vi "Lakeshore_372_write.vi"(5 "File reference":refnum<file>) -> ()   [LabVIEW 2019]
uses:
  Instrument_Setup.vi
  Global/Global Variables/Data_Display_global.vi
  Global/Global Variables/global.vi
panel:
  # "OFF"
  # "ON"
  # "OFF"
  # "ON"
  # "OFF"
  # "ON"
  # "OFF"
  # "ON"
  # "ON"
  # "OFF"
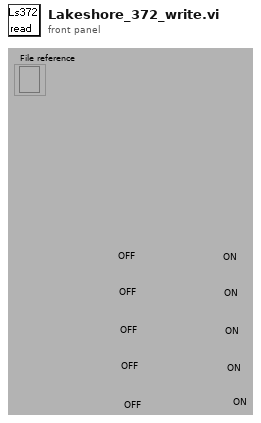
[diagram p1: front panel]
types:
  T1 = typedef "LS372-Cluster.ctl" = cluster{"Activate Tsweep":bool, "Setpoint - Manual":dbl, "Rate (K/min)":dbl, "Update Lakeshores":bool, "Still Heater":bool, "Still Power (mW)":dbl, "Manual Heater":bool, "Manual Heater  (mW) ":dbl, "Heater Range":dbl, "P (Gain)":dbl, "I (Reset)":dbl, "D (Rate)":dbl, "Heater Power (mW)":dbl, "MC Thermometer":u16, "MC Temperature":dbl, "LS372-T1":dbl, "LS372 -T2":dbl, "LS372-R1 ":dbl, "LS372-R2":dbl, "LS372-T3":dbl, "LS372-T4":dbl, "LS372-R3 ":dbl, "LS372-R4 \n\n\n\n":dbl, "LS372-T5":dbl, "LS372-T6":dbl, "LS372-R5":dbl, "LS372-R6 ":dbl, "Still Power ist":dbl, "Set Temperatur Sweep main":bool, "Setpoint ist":dbl, "Disable Heater":bool}
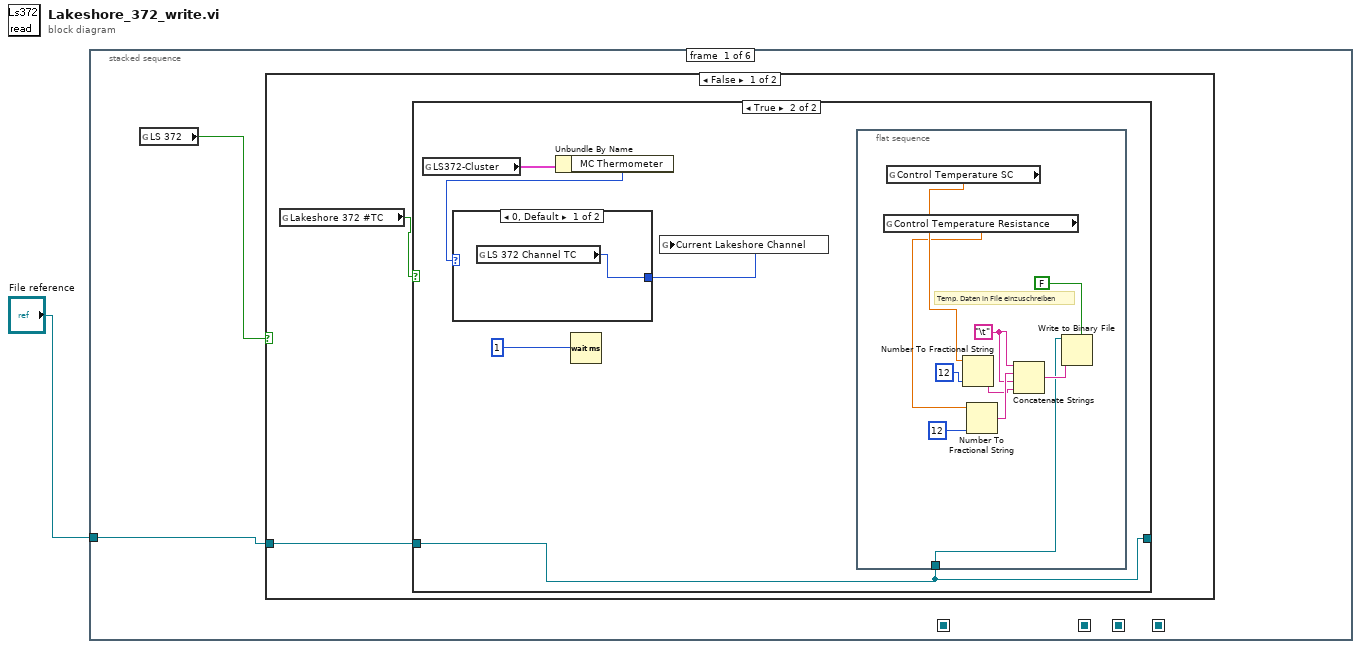
[diagram p0: block diagram]
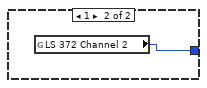
[diagram p3: hidden frame]
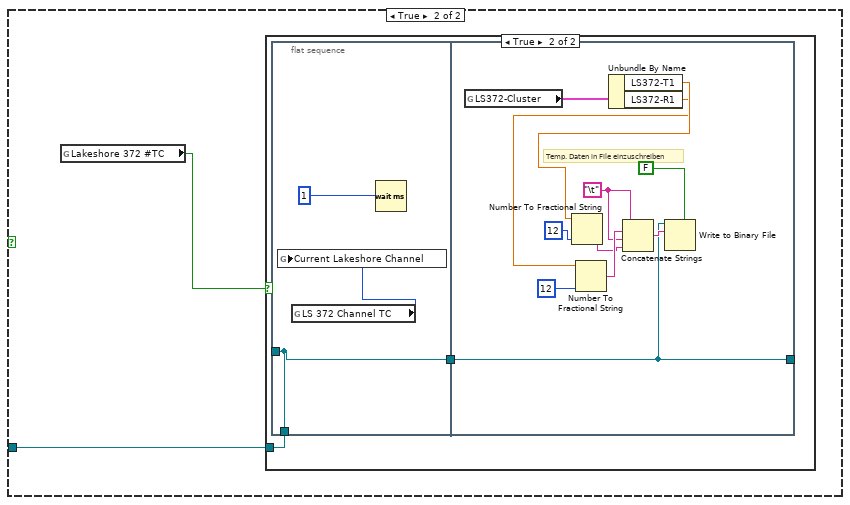
[diagram p4: hidden frame]
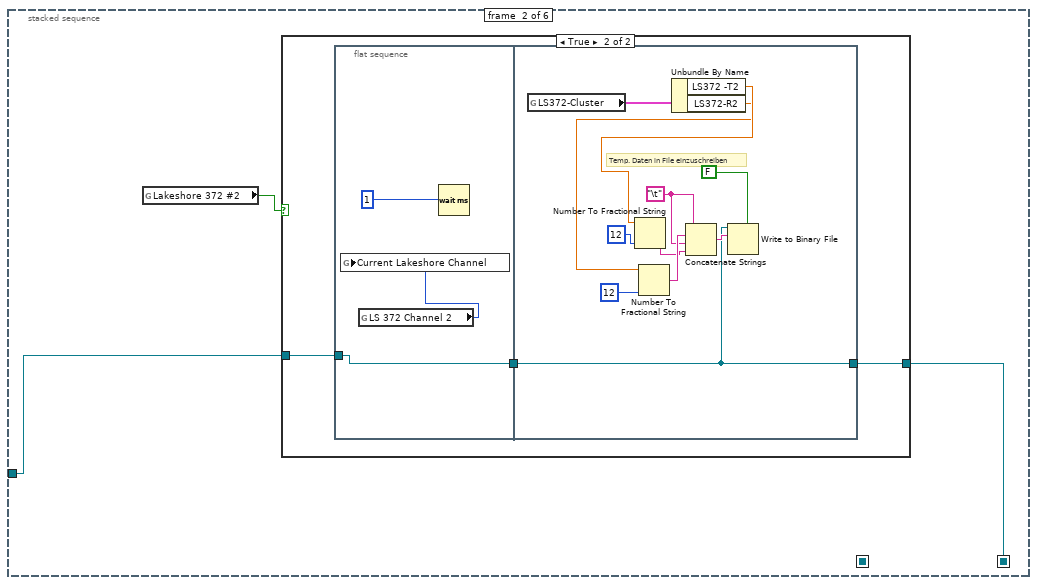
[diagram p6: hidden frame]
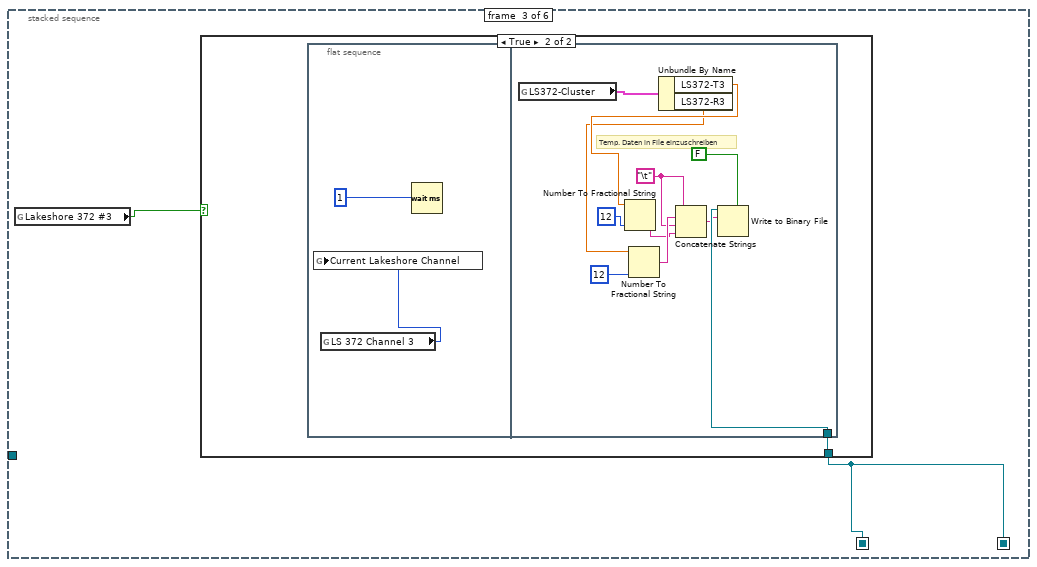
[diagram p8: hidden frame]
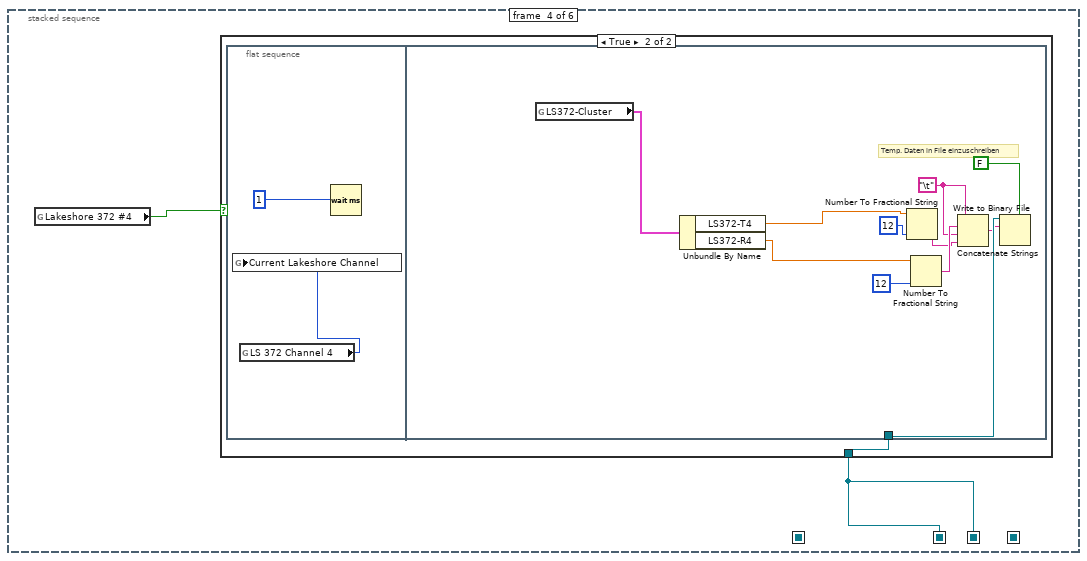
[diagram p10: hidden frame]
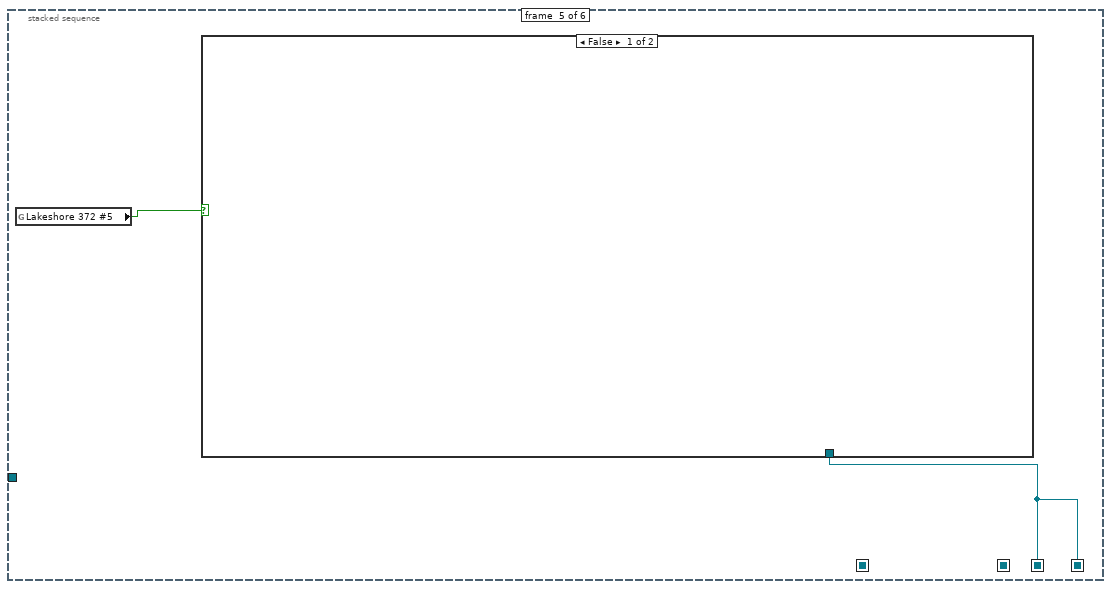
[diagram p12: hidden frame]
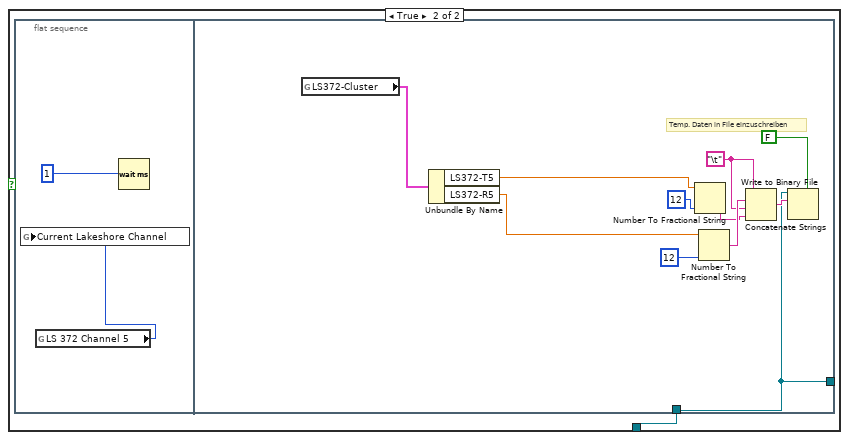
[diagram p13: hidden frame]
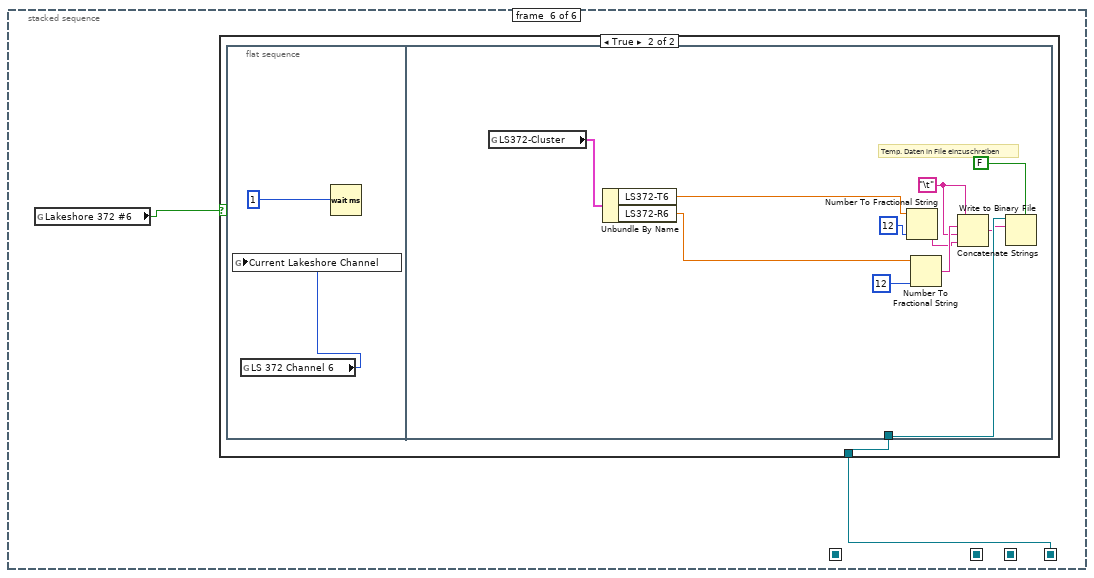
[diagram p14: hidden frame]
diagram:
  n1 = stacked-sequence {
    seq-local: [_ w42 _ _ _ _] -> [_ _ w63 w79 _ _]
    seq-local: [_ _ w63 _ _ _] -> [_ _ _ _ _ _]
    seq-local: [_ _ _ w79 _ _] -> [_ _ _ _ w95 _]
    seq-local: [_ _ _ _ w95 _] -> [_ _ _ _ _ w111]
    tunnel: "File reference" -> [w3 w43 _ _ _ _]
    frame #0 {
      n2 = global read "Instrument_Setup.vi" "LS 372"() -> (w2:bool)
      n3 = case shown="False" w2 {
        tunnel: w3 -> [w4 w24]
        frame False {
          n4 = global read "Instrument_Setup.vi" "Lakeshore 372 #TC"() -> (w5:bool)
          n5 = case shown="True" w5 {
            tunnel: w4 -> [w6 w7]
            tunnel: [w6 w7] -> _
            frame False {
            }
            frame True {
              n6 = global read "Data_Display_global.vi" "LS372-Cluster"() -> (w10:T1)
              n7 = Unbundle By Name(w10) -> ("MC Thermometer"=w9:u16)
              n8 = case shown="0, Default" w9 {
                tunnel: [w12 w13] -> w8
                frame 0, Default {
                  n9 = global read "Instrument_Setup.vi" "LS 372 Channel TC"() -> (w12:u16)
                }
                frame 1 {
                  n10 = global read "Instrument_Setup.vi" "LS 372 Channel 2"() -> (w13:u16)
                }
              }
              n11 = Wait (ms)(milliseconds to wait=1) -> ()  [unwired: 1 out]
              n12 = global write "global.vi" "Current Lakeshore Channel"(w8) -> ()
              n13 = flat-sequence {
                tunnel: w7 -> [w19]
                frame #0 {
                  w17 = "\t"
                  # "Temp. Daten in File einzuschreiben"
                  n14 = global read "Data_Display_global.vi" "Control Temperature Resistance"() -> (w14:dbl)
                  n15 = global read "Data_Display_global.vi" "Control Temperature SC"() -> (w15:dbl)
                  n16 = Number To Fractional String(number=w15, precision (6)=i16 12) -> (F-format string=w16:string)  [unwired: 2 in]
                  n17 = Number To Fractional String(number=w14, precision (6)=i16 12) -> (F-format string=w22:string)  [unwired: 2 in]
                  n18 = Concatenate Strings(w17, w22, w17, w16) -> (w23:string)
                  n19 = Write to Binary File ("Write File")(file (use dialog)=w19, data=w23, 5:FALSE ("prepend array or string size? (T)")) -> ()  [unwired: 3 in, 3 out]
                }
              }
            }
          }
        }
        frame True {
          n20 = global read "Instrument_Setup.vi" "Lakeshore 372 #TC"() -> (w25:bool)
          n21 = case shown="True" w25 {
            tunnel: w24 -> [_ w26]
            frame False {
            }
            frame True {
              n22 = flat-sequence {
                tunnel: [w28] -> _
                tunnel: [w28] -> w27
                tunnel: w26 -> [w28]
                tunnel: w27 -> [w34]
                tunnel: [w34] -> _
                frame #0 {
                  n23 = global read "Instrument_Setup.vi" "LS 372 Channel TC"() -> (w29:u16)
                  n24 = global write "global.vi" "Current Lakeshore Channel"(w29) -> ()
                  n25 = Wait (ms)(milliseconds to wait=1) -> ()  [unwired: 1 out]
                }
                frame #1 {
                  w37 = "\t"
                  # "Temp. Daten in File einzuschreiben"
                  n26 = global read "Data_Display_global.vi" "LS372-Cluster"() -> (w33:T1)
                  n27 = Unbundle By Name(w33) -> ("LS372-T1"=w32:dbl, "LS372-R1"=w31:dbl)
                  n28 = Number To Fractional String(number=w32, precision (6)=i16 12) -> (F-format string=w36:string)  [unwired: 2 in]
                  n29 = Number To Fractional String(number=w31, precision (6)=i16 12) -> (F-format string=w40:string)  [unwired: 2 in]
                  n30 = Concatenate Strings(w37, w40, w37, w36) -> (w35:string)
                  n31 = Write to Binary File ("Write File")(file (use dialog)=w34, data=w35, 5:FALSE ("prepend array or string size? (T)")) -> ()  [unwired: 3 in, 3 out]
                }
              }
            }
          }
        }
      }
    }
    frame #1 {
      n32 = global read "Instrument_Setup.vi" "Lakeshore 372 #2"() -> (w44:bool)
      n33 = case shown="True" w44 {
        tunnel: w43 -> [w45 w48]
        tunnel: [w45 w46] -> w42
        frame False {
        }
        frame True {
          n34 = flat-sequence {
            tunnel: w48 -> [w49]
            tunnel: [w49] -> w47
            tunnel: w47 -> [w55]
            tunnel: [w55] -> w46
            frame #0 {
              n35 = global read "Instrument_Setup.vi" "LS 372 Channel 2"() -> (w50:u16)
              n36 = global write "global.vi" "Current Lakeshore Channel"(w50) -> ()
              n37 = Wait (ms)(milliseconds to wait=1) -> ()  [unwired: 1 out]
            }
            frame #1 {
              w58 = "\t"
              # "Temp. Daten in File einzuschreiben"
              n38 = global read "Data_Display_global.vi" "LS372-Cluster"() -> (w54:T1)
              n39 = Unbundle By Name(w54) -> ("LS372 -T2"=w53:dbl, "LS372-R2"=w52:dbl)
              n40 = Number To Fractional String(number=w53, precision (6)=i16 12) -> (F-format string=w57:string)  [unwired: 2 in]
              n41 = Number To Fractional String(number=w52, precision (6)=i16 12) -> (F-format string=w61:string)  [unwired: 2 in]
              n42 = Concatenate Strings(w58, w61, w58, w57) -> (w56:string)
              n43 = Write to Binary File ("Write File")(file (use dialog)=w55, data=w56, 5:FALSE ("prepend array or string size? (T)")) -> ()  [unwired: 3 in, 3 out]
            }
          }
        }
      }
    }
    frame #2 {
      n44 = global read "Instrument_Setup.vi" "Lakeshore 372 #3"() -> (w64:bool)
      n45 = case shown="True" w64 {
        tunnel: w63 -> [_ w65]
        frame False {
        }
        frame True {
          n46 = flat-sequence {
            tunnel: w65 -> [w77]
            frame #0 {
              n47 = global read "Instrument_Setup.vi" "LS 372 Channel 3"() -> (w66:u16)
              n48 = global write "global.vi" "Current Lakeshore Channel"(w66) -> ()
              n49 = Wait (ms)(milliseconds to wait=1) -> ()  [unwired: 1 out]
            }
            frame #1 {
              w73 = "\t"
              # "Temp. Daten in File einzuschreiben"
              n50 = global read "Data_Display_global.vi" "LS372-Cluster"() -> (w70:T1)
              n51 = Unbundle By Name(w70) -> ("LS372-T3"=w69:dbl, "LS372-R3"=w68:dbl)
              n52 = Number To Fractional String(number=w69, precision (6)=i16 12) -> (F-format string=w72:string)  [unwired: 2 in]
              n53 = Number To Fractional String(number=w68, precision (6)=i16 12) -> (F-format string=w76:string)  [unwired: 2 in]
              n54 = Concatenate Strings(w73, w76, w73, w72) -> (w71:string)
              n55 = Write to Binary File ("Write File")(file (use dialog)=w77, data=w71, 5:FALSE ("prepend array or string size? (T)")) -> ()  [unwired: 3 in, 3 out]
            }
          }
        }
      }
    }
    frame #3 {
      n56 = global read "Instrument_Setup.vi" "Lakeshore 372 #4"() -> (w80:bool)
      n57 = case shown="True" w80 {
        tunnel: w79 -> [_ w81]
        frame False {
        }
        frame True {
          n58 = flat-sequence {
            tunnel: w81 -> [w93]
            frame #0 {
              n59 = global read "Instrument_Setup.vi" "LS 372 Channel 4"() -> (w82:u16)
              n60 = global write "global.vi" "Current Lakeshore Channel"(w82) -> ()
              n61 = Wait (ms)(milliseconds to wait=1) -> ()  [unwired: 1 out]
            }
            frame #1 {
              w89 = "\t"
              # "Temp. Daten in File einzuschreiben"
              n62 = global read "Data_Display_global.vi" "LS372-Cluster"() -> (w86:T1)
              n63 = Unbundle By Name(w86) -> ("LS372-T4"=w85:dbl, "LS372-R4"=w84:dbl)
              n64 = Number To Fractional String(number=w85, precision (6)=i16 12) -> (F-format string=w88:string)  [unwired: 2 in]
              n65 = Number To Fractional String(number=w84, precision (6)=i16 12) -> (F-format string=w92:string)  [unwired: 2 in]
              n66 = Concatenate Strings(w89, w92, w89, w88) -> (w87:string)
              n67 = Write to Binary File ("Write File")(file (use dialog)=w93, data=w87, 5:FALSE ("prepend array or string size? (T)")) -> ()  [unwired: 3 in, 3 out]
            }
          }
        }
      }
    }
    frame #4 {
      n68 = global read "Instrument_Setup.vi" "Lakeshore 372 #5"() -> (w96:bool)
      n69 = case shown="False" w96 {
        tunnel: w95 -> [_ w97]
        frame False {
        }
        frame True {
          n70 = flat-sequence {
            tunnel: w97 -> [w100]
            tunnel: [w100] -> _
            frame #0 {
              n71 = global read "Instrument_Setup.vi" "LS 372 Channel 5"() -> (w98:u16)
              n72 = global write "global.vi" "Current Lakeshore Channel"(w98) -> ()
              n73 = Wait (ms)(milliseconds to wait=1) -> ()  [unwired: 1 out]
            }
            frame #1 {
              w106 = "\t"
              # "Temp. Daten in File einzuschreiben"
              n74 = global read "Data_Display_global.vi" "LS372-Cluster"() -> (w103:T1)
              n75 = Unbundle By Name(w103) -> ("LS372-T5"=w102:dbl, "LS372-R5"=w101:dbl)
              n76 = Number To Fractional String(number=w102, precision (6)=i16 12) -> (F-format string=w105:string)  [unwired: 2 in]
              n77 = Number To Fractional String(number=w101, precision (6)=i16 12) -> (F-format string=w109:string)  [unwired: 2 in]
              n78 = Concatenate Strings(w106, w109, w106, w105) -> (w104:string)
              n79 = Write to Binary File ("Write File")(file (use dialog)=w100, data=w104, 5:FALSE ("prepend array or string size? (T)")) -> ()  [unwired: 3 in, 3 out]
            }
          }
        }
      }
    }
    frame #5 {
      n80 = global read "Instrument_Setup.vi" "Lakeshore 372 #6"() -> (w112:bool)
      n81 = case shown="True" w112 {
        tunnel: w111 -> [_ w113]
        frame False {
        }
        frame True {
          n82 = flat-sequence {
            tunnel: w113 -> [w125]
            frame #0 {
              n83 = global read "Instrument_Setup.vi" "LS 372 Channel 6"() -> (w114:u16)
              n84 = global write "global.vi" "Current Lakeshore Channel"(w114) -> ()
              n85 = Wait (ms)(milliseconds to wait=1) -> ()  [unwired: 1 out]
            }
            frame #1 {
              w121 = "\t"
              # "Temp. Daten in File einzuschreiben"
              n86 = global read "Data_Display_global.vi" "LS372-Cluster"() -> (w118:T1)
              n87 = Unbundle By Name(w118) -> ("LS372-T6"=w117:dbl, "LS372-R6"=w116:dbl)
              n88 = Number To Fractional String(number=w117, precision (6)=i16 12) -> (F-format string=w120:string)  [unwired: 2 in]
              n89 = Number To Fractional String(number=w116, precision (6)=i16 12) -> (F-format string=w124:string)  [unwired: 2 in]
              n90 = Concatenate Strings(w121, w124, w121, w120) -> (w119:string)
              n91 = Write to Binary File ("Write File")(file (use dialog)=w125, data=w119, 5:FALSE ("prepend array or string size? (T)")) -> ()  [unwired: 3 in, 3 out]
            }
          }
        }
      }
    }
  }
